vi "Get Build Specification Name.vi"(8 "error in (no error)":errorcluster, 11 "NI_AB_API_EXE in":refnum<class "NI_AB_API_EXE.lvclass">) -> (0 "error out":errorcluster, 2 "Build Specification Name":string, 3 "NI_AB_API_EXE out":refnum<class "NI_AB_API_EXE.lvclass">)   [LabVIEW 2020, in "NI_AB_API_EXE.lvclass"]
uses:
  <vilib>/AppBuilder/AB_API/EXE/NI_AB_API_EXE.lvclass
  <vilib>/AppBuilder/AB_API/EXE/NI_AB_API_EXE.lvclass/NI_AB_API_EXE.ctl
  <vilib>/AppBuilder/AB_API/Application/NI_AB_API_Application.lvclass
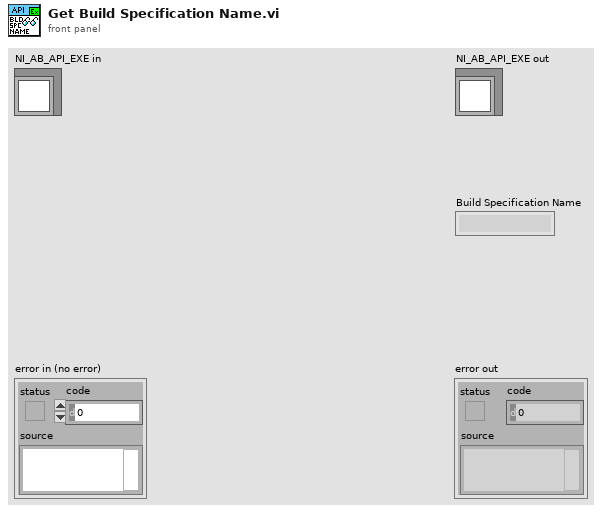
[diagram p1: front panel]
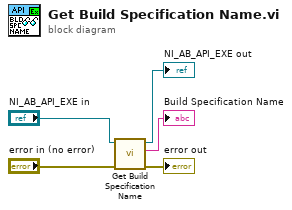
[diagram p0: block diagram]
diagram:
  n1 = call-parent "Get Build Specification Name.vi"("error in (no error)"="error in (no error)", "NI_AB_API_Build in"="NI_AB_API_EXE in") -> ("error out"=→"error out":errorcluster, "Build Specification Name"=→"Build Specification Name":string, "NI_AB_API_Build out"=→"NI_AB_API_EXE out":refnum<class "NI_AB_API_EXE.lvclass">)  [unwired: 7 in]
